vi "HJ212-2017.vi"(8 "error in (no error)":errorcluster caption="错误输入（无错误）", 10 "PWD？":bool, 11 "数据段":T1) -> (0 "error out":errorcluster caption="错误输出", 2 "通讯包字符串":string, 3 "通讯包":T2={"包头（2）"="##", "数据段长度（4）"="", "数据段"="", "CRC校验"="", "包尾"=""})   [LabVIEW 2016, in "潮位站数据传输.lvlib" / "HJ212.lvclass"]
uses:
  HJ212.lvclass
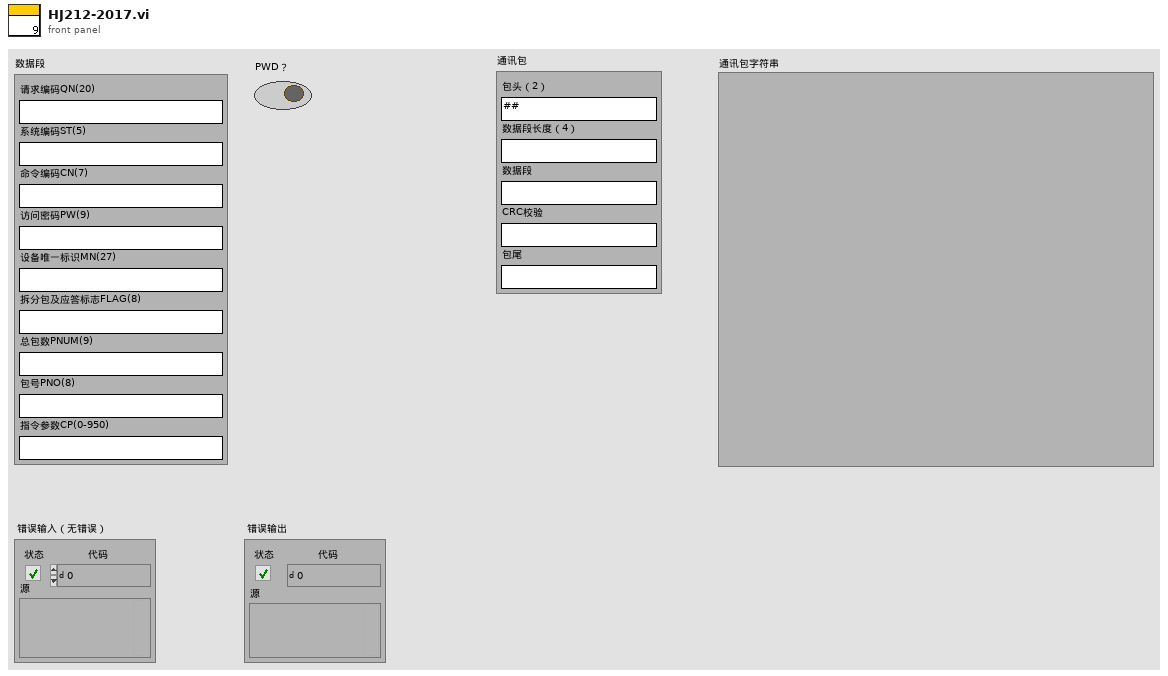
[diagram p1: front panel]
types:
  T1 = cluster{"请求编码QN(20)":string, "系统编码ST(5)":string, "命令编码CN(7)":string, "访问密码PW(9)":string, "设备唯一标识MN(27)":string, "拆分包及应答标志FLAG(8)":string, "总包数PNUM(9)":string, "包号PNO(8)":string, "指令参数CP(0-950)":string}
  T2 = cluster{"包头（2）":string, "数据段长度（4）":string, "数据段":string, "CRC校验":string, "包尾":string}
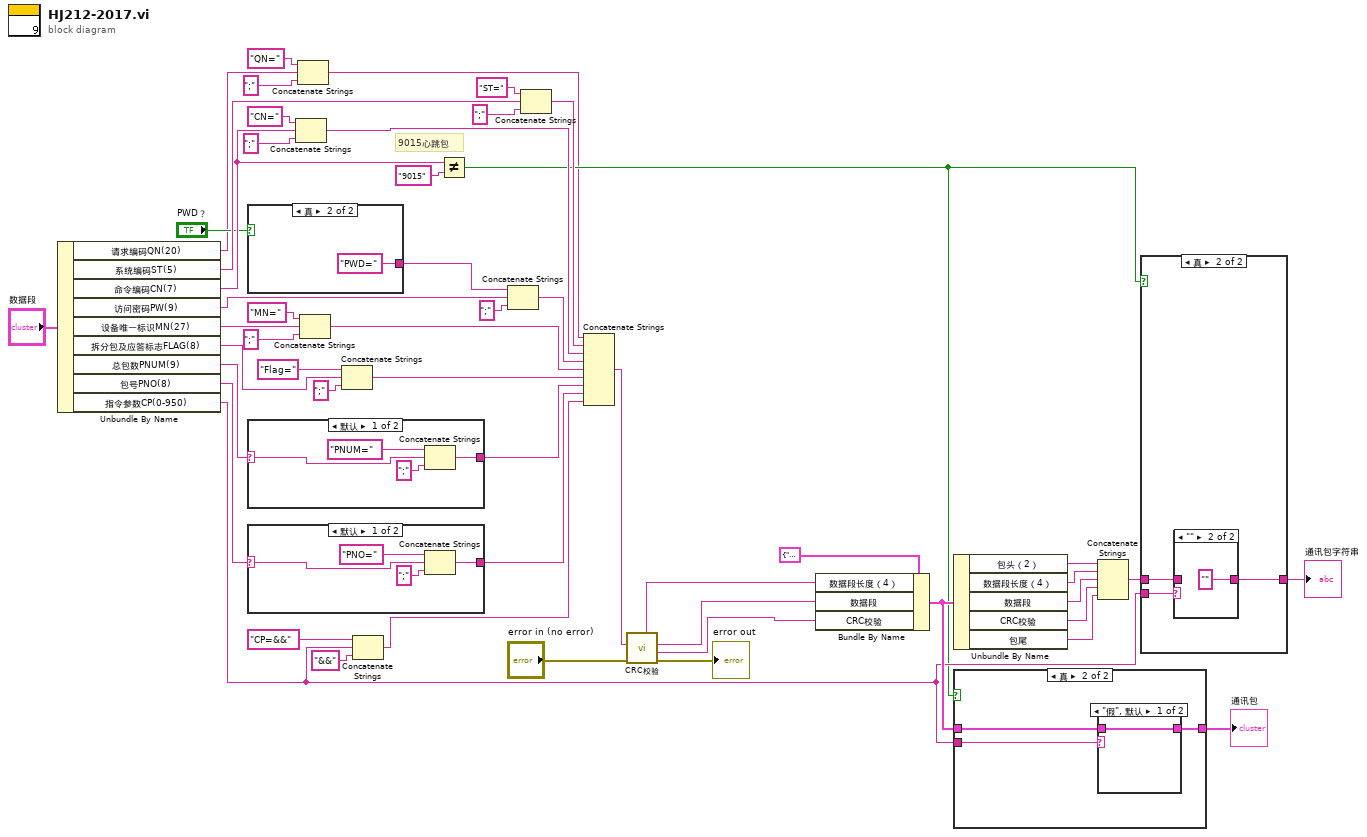
[diagram p0: block diagram]
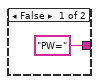
[diagram p2: hidden frame]
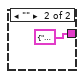
[diagram p6: hidden frame]
diagram:
  # "9015心跳包"
  n1 = Unbundle By Name("数据段") -> ("请求编码QN(20)"=w14:string, "系统编码ST(5)"=w51:string, "命令编码CN(7)"=w19:string, "访问密码PW(9)"=w47:string, "设备唯一标识MN(27)"=w45:string, "拆分包及应答标志FLAG(8)"=w12:string, "总包数PNUM(9)"=w37:string, "包号PNO(8)"=w35:string, "指令参数CP(0-950)"=w20:string)
  n2 = case shown="真" "PWD？" {
    tunnel: ["PW=" ("字符串") "PWD=" ("字符串")] -> w15
    frame False {
    }
    frame True {
    }
  }
  n3 = case shown="默认" w37 {
    selector: w37 -> [w57 w59]
    tunnel: [w55 w59] -> w36
    frame Default {
      n4 = Concatenate Strings("PNUM=" ("字符串"), w57, ";" ("字符串")) -> (w55:string)
    }
    frame "" {
    }
  }
  n5 = case shown="默认" w35 {
    selector: w35 -> [w62 w64]
    tunnel: [w60 w64] -> w34
    frame Default {
      n6 = Concatenate Strings("PNO=" ("字符串"), w62, ";" ("字符串")) -> (w60:string)
    }
    frame "" {
    }
  }
  n7 = Concatenate Strings("CN=" ("字符串"), w19, ";" ("字符串")) -> (w41:string)
  n8 = Concatenate Strings("QN=" ("字符串"), w14, ";" ("字符串")) -> (w13:string)
  n9 = Concatenate Strings("MN=" ("字符串"), w45, ";" ("字符串")) -> (w39:string)
  n10 = Concatenate Strings("Flag=" ("字符串"), w12, ";" ("字符串")) -> (w11:string)
  n11 = Concatenate Strings("CP=&&" ("字符串"), w20, "&&" ("字符串")) -> (w31:string)
  n12 = Not Equal?(x=w19, y="9015") -> (x != y?=w17:bool)
  n13 = Concatenate Strings(w15, w47, ";" ("字符串")) -> (w40:string)
  n14 = Concatenate Strings("ST=" ("字符串"), w51, ";" ("字符串")) -> (w42:string)
  n15 = Concatenate Strings(w13, w42, w41, w40, w39, w11, w36, w34, w31) -> (w6:string)
  n16 = call "CRC校验.vi"("error in (no error)"="error in (no error)", "puchMsg"=w6) -> ("error out"=→"error out":errorcluster, "CRC校验"=w3:string, "数据段"=w4:string, "数据段长度"=w5:string)  [unwired: 6 in]
  n17 = Bundle By Name(cluster=T2 {"包头（2）"="##", "数据段长度（4）"="", "数据段"="", "CRC校验"="", "包尾"="\r\n"} ("通讯包"), "数据段长度（4）"=w5, "数据段"=w4, "CRC校验"=w3) -> (w22:T2)
  n18 = Unbundle By Name(w22) -> ("包头（2）"=w29:string, "数据段长度（4）"=w28:string, "数据段"=w27:string, "CRC校验"=w26:string, "包尾"=w25:string)
  n19 = case shown="真" w17 {
    tunnel: w22 -> [w65 w68]
    tunnel: [w65 w67] -> w21
    tunnel: w20 -> [_ w66]
    frame False {
    }
    frame True {
      n20 = case shown="\"假\", 默认" w66 {
        tunnel: [w69 T2 {"包头（2）"="", "数据段长度（4）"="", "数据段"="", "CRC校验"="", "包尾"=""} ("通讯包")] -> w67
        tunnel: w68 -> [w69 _]
        frame "假", Default {
        }
        frame "" {
        }
      }
    }
  }
  "通讯包" <- w21
  n21 = Concatenate Strings(w29, w28, w27, w26, w25) -> (w24:string)
  n22 = case shown="真" w17 {
    tunnel: w24 -> [w71 w74]
    tunnel: [w71 w73] -> w23
    tunnel: w20 -> [_ w72]
    frame False {
    }
    frame True {
      n23 = case shown="\"\"" w72 {
        tunnel: [w75 ""] -> w73
        tunnel: w74 -> [w75 _]
        frame "假", Default {
        }
        frame "" {
        }
      }
    }
  }
  "通讯包字符串" <- w23
